vi "差分全体均值重建数据准备.vi"(0 "关联成像原理":dbl, 5 "重建方法":dbl, 7 "优化算法":dbl, 9 "光源散斑簇":T2, 11 "图像簇":T1) -> (4 "照射结果求和数组":dbl[](array[numeric]), 6 "照射结果求和均值":dbl)   [LabVIEW 2018]
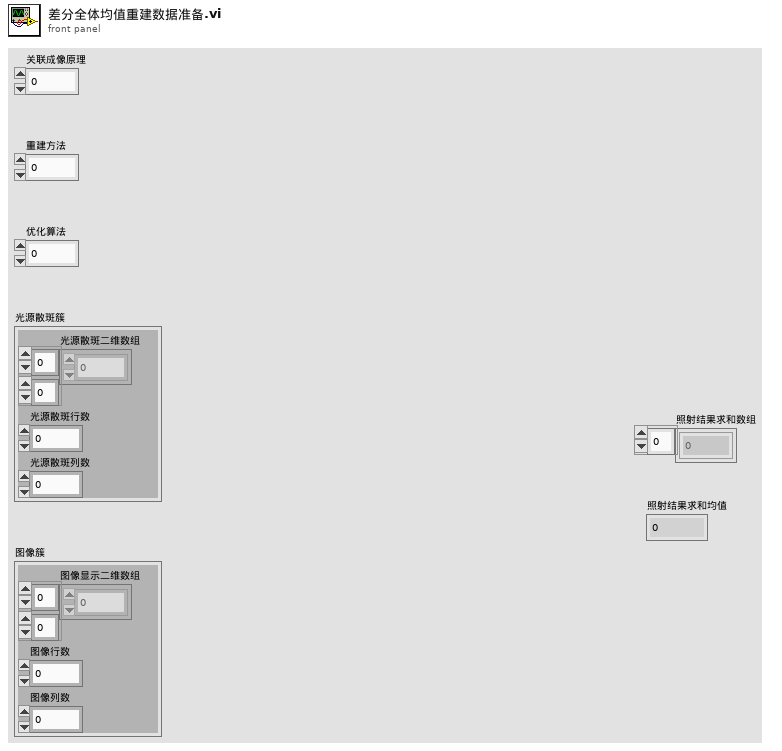
[diagram p1: front panel]
types:
  T1 = cluster{"图像显示二维数组":dbl[][], "图像行数":i32, "图像列数":i32}
  T2 = cluster{"光源散斑二维数组":dbl[][], "光源散斑行数":i32, "光源散斑列数":i32}
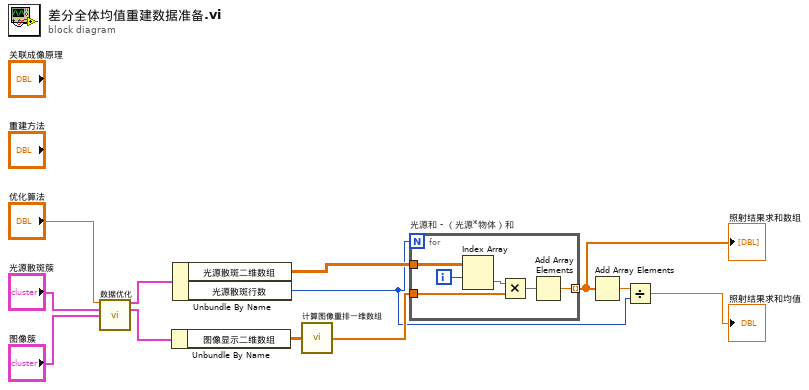
[diagram p0: block diagram]
diagram:
  n1 = call "数据优化.vi"("优化算法"="优化算法", "光源散斑簇"="光源散斑簇", "图像簇"="图像簇") -> ("优化光源散斑簇"=w2:T2, "优化图像簇"=w1:T1)  [unwired: 11 in]
  n2 = Unbundle By Name(w1) -> ("图像显示二维数组"=w12:dbl[][])
  n3 = Unbundle By Name(w2) -> ("光源散斑二维数组"=w8:dbl[][], "光源散斑行数"=w6:i32)
  n4 = call "计算图像重排一维数组.vi"("图像二维数组"=w12) -> ("图像重排一维数组"=w7:dbl[])
  n5 = for "光源和 - （光源*物体）和" {
    N: w6 -> [_]
    tunnel: w8 -> [w18]
    tunnel: w7 -> [w17]
    tunnel: [w14] -> w9 mode=indexing
    i -> [w13]
    n6 = Index Array(array=w18, index (row)=w13) -> (element=w15:dbl[])  [unwired: 1 in]
    n7 = Multiply(x=w15, y=w17) -> (x*y=w16:dbl[])
    n8 = Add Array Elements(numeric array=w16) -> (sum=w14:dbl)
  }
  "照射结果求和数组" <- w9
  n9 = Add Array Elements(numeric array=w9) -> (sum=w11:dbl)
  n10 = Divide(x=w11, y=w6) -> (x/y=→"照射结果求和均值":dbl)
